vi "Generator_11.vi"(4 "pulser ON/OFF":bool, 5 "remote echo":bool, 7 "internal trigger":bool, 8 "Puls mode":u16(ring) items=["Half cycle positive", "Half cycle negegative", "Full cycle positive", "Full cycle negative"], 9 "high gain":bool) -> (0 "Command_ str":string)   [LabVIEW 2022 SP3]
panel:
  out "Command_ str 2":string
  out "hex str":string
  out "decimal":i32
  out "binary str":string
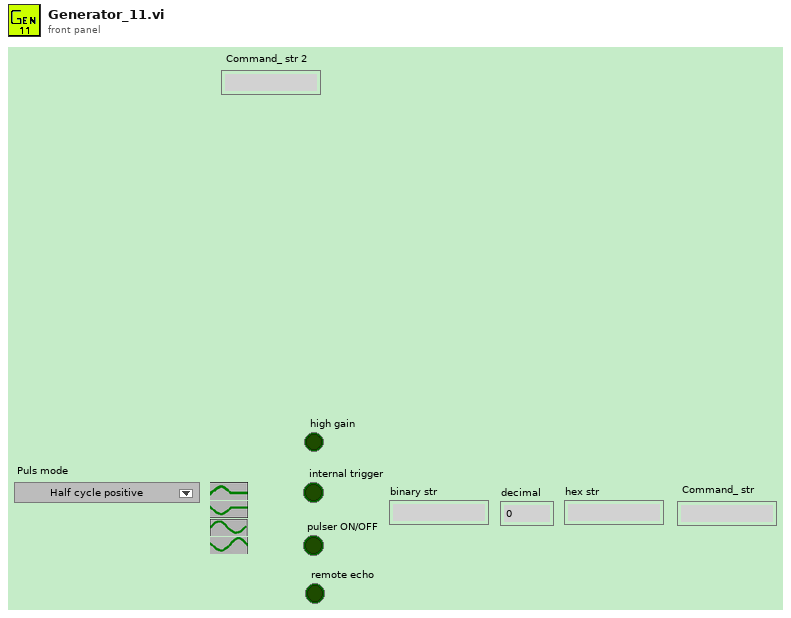
[diagram p1: front panel]
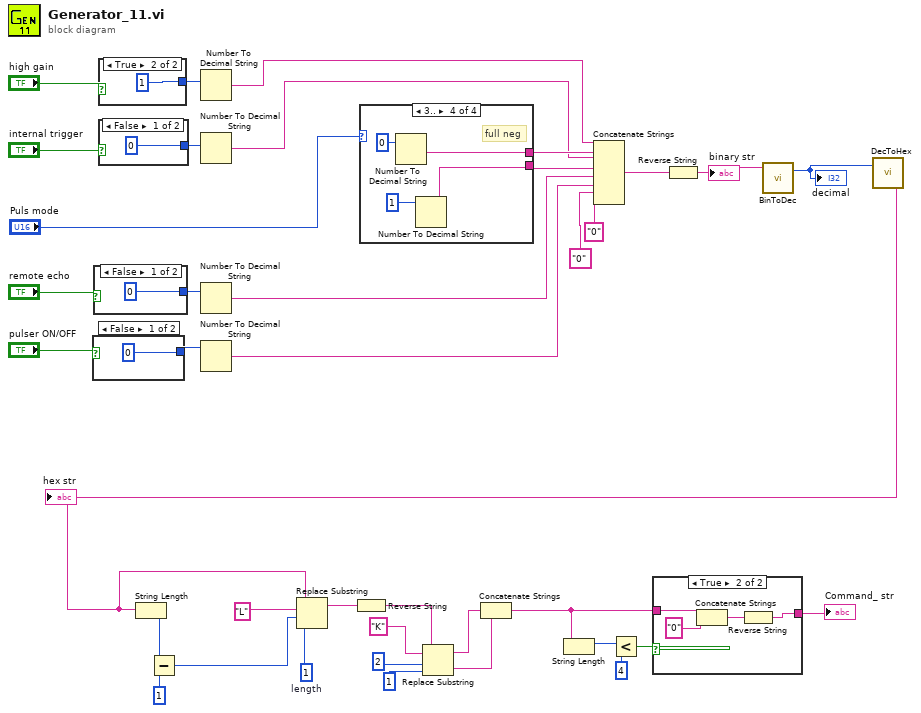
[diagram p0: block diagram]
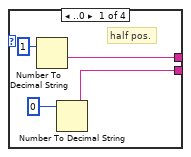
[diagram p2: hidden frame]
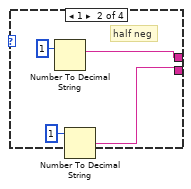
[diagram p3: hidden frame]
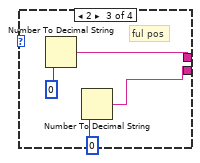
[diagram p4: hidden frame]
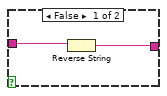
[diagram p5: hidden frame]
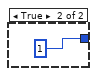
[diagram p6: hidden frame]
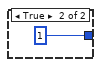
[diagram p7: hidden frame]
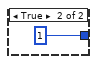
[diagram p8: hidden frame]
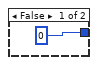
[diagram p9: hidden frame]
diagram:
  w28 = 1  # length
  n1 = case shown="False" "pulser ON/OFF" {
    tunnel: [0 1] -> w34
    frame False {
    }
    frame True {
    }
  }
  n2 = case shown="False" "remote echo" {
    tunnel: [0 1] -> w32
    frame False {
    }
    frame True {
    }
  }
  n3 = case shown="True" "high gain" {
    tunnel: [0 1] -> w31
    frame False {
    }
    frame True {
    }
  }
  n4 = case shown="False" "internal trigger" {
    tunnel: [0 1] -> w37
    frame False {
    }
    frame True {
    }
  }
  n5 = Number To Decimal String(number=w31) -> (decimal integer string=w7:string)  [unwired: 1 out]
  n6 = Number To Decimal String(number=w37) -> (decimal integer string=w6:string)  [unwired: 1 out]
  n7 = Number To Decimal String(number=w32) -> (decimal integer string=w3:string)  [unwired: 1 out]
  n8 = Number To Decimal String(number=w34) -> (decimal integer string=w2:string)  [unwired: 1 out]
  n9 = case shown="3.." "Puls mode" {
    tunnel: [w48 w51 w55 w59] -> w10
    tunnel: [w47 w52 w56 w60] -> w9
    frame ..0 {
      # "half pos."
      n10 = Number To Decimal String(number=1) -> (decimal integer string=w47:string)  [unwired: 1 out]
      n11 = Number To Decimal String(number=0) -> (decimal integer string=w48:string)  [unwired: 1 out]
    }
    frame 1 {
      (unwired) 4
      (unwired) 1
      (unwired) 2
      (unwired) "K"
      (unwired) "L"
      (unwired) 1
      (unwired) 1  # length
      # "half neg"
      n12 = Number To Decimal String(number=1) -> (decimal integer string=w52:string)  [unwired: 1 out]
      n13 = Number To Decimal String(number=1) -> (decimal integer string=w51:string)  [unwired: 1 out]
    }
    frame 2 {
      # "ful pos"
      n14 = Number To Decimal String(number=0) -> (decimal integer string=w56:string)  [unwired: 1 out]
      n15 = Number To Decimal String(number=0) -> (decimal integer string=w55:string)  [unwired: 1 out]
    }
    frame 3.. {
      # "full neg"
      n16 = Number To Decimal String(number=0) -> (decimal integer string=w60:string)  [unwired: 1 out]
      n17 = Number To Decimal String(number=1) -> (decimal integer string=w59:string)  [unwired: 1 out]
    }
  }
  n18 = Concatenate Strings(w7, w9, w6, w10, w3, w2, "0", "0") -> (w11:string)
  n19 = Reverse String(1:w11) -> (0:w8:string)
  "binary str" <- w8
  n20 = call "BinToDec.vi"("Number String (0010)"=w8) -> ("Converted number (decimal)"=w30:i32)  [unwired: 2 in, 1 out]
  "decimal" <- w30
  n21 = call "DecToHex.vi"("Decimal . Decimal Representation"=w30) -> ("HEX . HEX representation"=w29:string)  [unwired: 1 out]
  "hex str" <- w29
  n22 = String Length(string=w29) -> (length=w26:i32)
  n23 = Subtract(x=w26, y=1) -> (x-y=w13:i32)
  n24 = Replace Substring(2:w28, 3:w13, 4:"L", 5:w29) -> (1:w25:string)  [unwired: 1 out]
  n25 = Reverse String(1:w25) -> (0:w24:string)
  n26 = Replace Substring(2:1, 3:2, 4:"K", 5:w24) -> (0:w19:string, 1:w20:string)
  n27 = Concatenate Strings(w20, w19) -> (w16:string)
  n28 = String Length(string=w16) -> (length=w18:i32)
  n29 = Less?(x=w18, y=4) -> (x < y?=w15:bool)
  n30 = case shown="True" w15 {
    tunnel: w16 -> [w64 w67]
    tunnel: [w63 w65] -> w14
    frame False {
      n31 = Reverse String(1:w64) -> (0:w63:string)
    }
    frame True {
      n32 = Concatenate Strings(w67, "0") -> (w66:string)
      n33 = Reverse String(1:w66) -> (0:w65:string)
    }
  }
  "Command_ str" <- w14
